vi "AlliGator Find & Plot Zero-Crossing Position v2.vi"(6 "Shift":dbl, 8 "Error In":errorcluster, 9 "Time Stamp":dbl, 10 "Lifetime Graph":refnum<vi>, 11 "Decay Graph":refnum<vi>) -> (0 "Error Out":errorcluster, 3 "Zero Position":dbl)   [LabVIEW 2021, in "AlliGator Decay Analysis.lvlib" / "AlliGator Decay Preprocessing.lvlib"]
doc: "Finds the zero-crossing location for the last decay in the <B>Decay Graph</B> using the provided <B>Shift</B> and adds it to the last plot in the <B>Lifetime & Other Parameters Graph</B>."
uses:
  AlliGator Decay Preprocessing.lvlib
  Graphs/XY Graph/XY Graph Add-Ons.lvlib
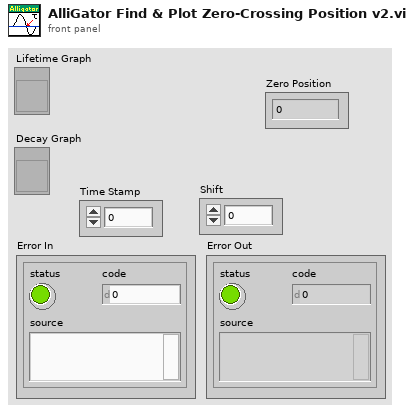
[diagram p1: front panel]
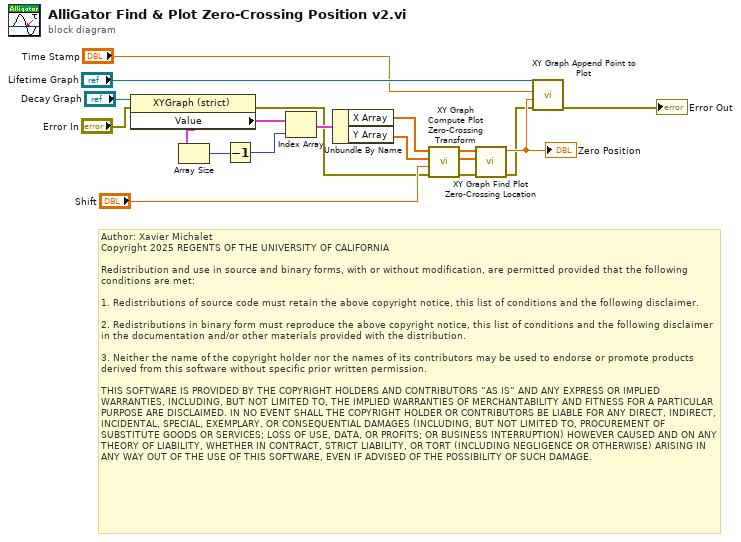
[diagram p0: block diagram]
diagram:
  # "Author: Xavier Michalet\nCopyright 2025 REGENTS OF THE UNIVERSITY OF CALIFORNIA\n\nRedistribution and use in source and binary forms, with or without modification, are permitted provided that the following conditions are met:\n\n1. Redistributions of source code must retain the above copyright notice, this list of conditions and the following disclaimer.\n\n2. Redistributions in binary form must reproduce the above copyright notice, this list of conditions and the following disclaimer in the documentation and/or other materials provided with the distribution.\n\n3. Neither the name of the copyright holder nor the names of its contributors may be used to endorse or promote products derived from this software without specific prior written permission.\n\nTHIS SOFTWARE IS PROVIDED BY THE COPYRIGHT HOLDERS AND CONTRIBUTORS “AS IS” AND ANY EXPRESS OR IMPLIED WARRANTIES, INCLUDING, BUT NOT LIMITED TO, THE IMPLIED WARRANTIES OF MERCHANTABILITY AND FITNESS FOR A PARTICULAR PURPOSE ARE DISCLAIMED. IN NO EVENT SHALL THE COPYRIGHT HOLDER OR CONTRIBUTORS BE LIABLE FOR ANY DIRECT, INDIRECT, INCIDENTAL, SPECIAL, EXEMPLARY, OR CONSEQUENTIAL DAMAGES (INCLUDING, BUT NOT LIMITED TO, PROCUREMENT OF SUBSTITUTE GOODS OR SERVICES; LOSS OF USE, DATA, OR PROFITS; OR BUSINESS INTERRUPTION) HOWEVER CAUSED AND ON ANY THEORY OF LIABILITY, WHETHER IN CONTRACT, STRICT LIABILITY, OR TORT (INCLUDING NEGLIGENCE OR OTHERWISE) ARISING IN ANY WAY OUT OF THE USE OF THIS SOFTWARE, EVEN IF ADVISED OF THE POSSIBILITY OF SUCH DAMAGE."
  n1 = property class="XYGraph (strict)"(reference="Decay Graph", error in="Error In") -> (error out=w2:errorcluster, "Value"=w16:cluster{"X Array":dbl[], "Y Array":dbl[]}[])  [unwired: 1 out]
  n2 = Array Size(array=w16) -> (size(s)=w15:i32)
  n3 = Decrement(x=w15) -> (x-1=w10:i32)
  n4 = Index Array(array=w16, index=w10) -> (element=w14:cluster{"X Array":dbl[], "Y Array":dbl[]})
  n5 = Unbundle By Name(w14) -> ("X Array"=w7:dbl[], "Y Array"=w8:dbl[])
  n6 = call "XY Graph Compute Plot Zero-Crossing Transform.vi"("Error In"=w2, "Shift"="Shift", "IRF Array in"=w8, "t Array in"=w7) -> ("Error Out"=w3:errorcluster, "ZC IRF Array out"=w5:dbl[], "t Array (dup) out"=w6:dbl[])  [unwired: 5 in]
  n7 = call "XY Graph Find Plot Zero-Crossing Location.vi"("Error In"=w3, "Y Array"=w5, "X Array"=w6) -> ("Error Out"=w1:errorcluster, "Zero Crossing Location"=w12:dbl)  [unwired: 6 in, 1 out]
  "Zero Position" <- w12
  n8 = call "XY Graph Append Point to Plot.vi"("error in (no error)"=w1, "y"=w12, "x"="Time Stamp", "XYGraph in"="Lifetime Graph") -> ("error out"=→"Error Out":errorcluster)  [unwired: 4 in, 3 out]
